vi "Read Encaspulation LEIN Header.vi"(7 "LEIN encapsulated Data and header":u8[](array[numeric]), 11 "error in (no error)":errorcluster) -> (4 "ACK":bool, 6 "SID":u8, 8 "CMD":u8, 10 "LEN":u8, 13 "Data":u8[](array[numeric]), 14 "Data len":i32, 15 "error out":errorcluster)   [LabVIEW 2011]
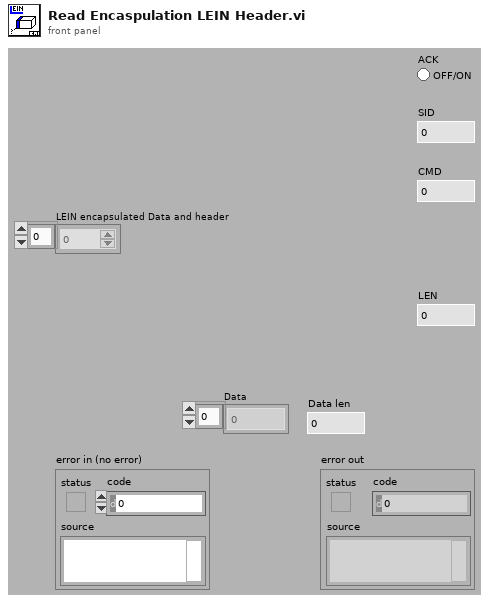
[diagram p1: front panel]
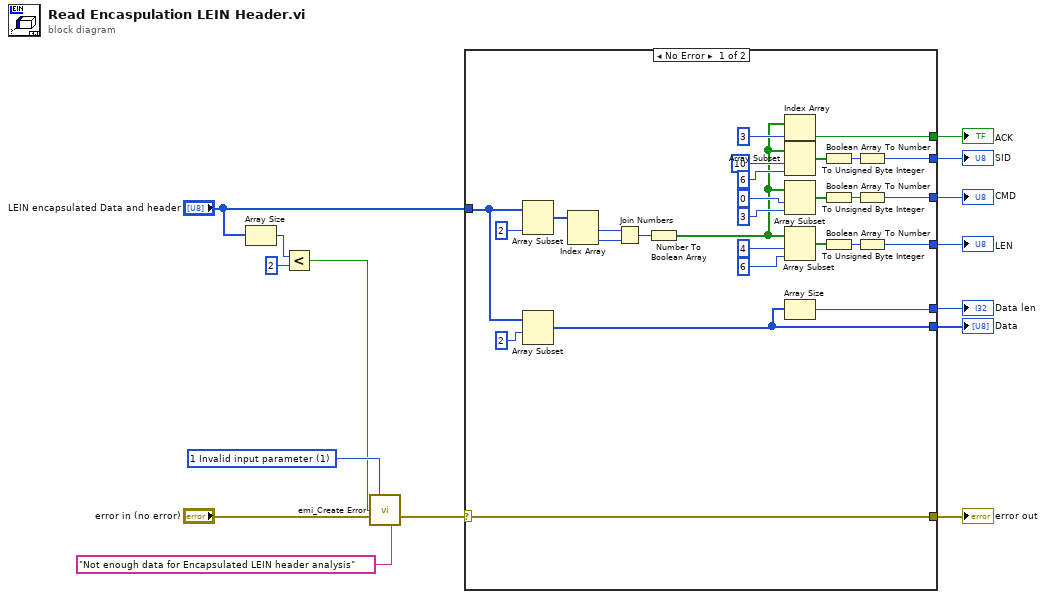
[diagram p0: block diagram]
diagram:
  w5 = 1 items=["0 No Error"=0, "1 Invalid input parameter"=1, "6 Generic file IO "=6, "7 File not Found"=7, "35 Generic Pring Error"=35, "37 Device not Found"=37, "39 Device Unit Error"=39, "40 Could fot Open Device"=40, "42 Generic Error"=42, "52 Unknown Message"=52, "98 Bad File type"=98, "99 Bad File Version"=99, "100 Bad Data in File"=100, "1018 Unspecefied Error"=1018, "1041 Incorrect Password"=1041, "1043 Feature not in this version"=1043, "1109 Unsuported Data type"=1109, "1444 Did not close sucessfully"=1444] ("Error Code")
  n1 = Array Size(array="LEIN encapsulated Data and header") -> (size(s)=w3:i32)
  n2 = Less?(x=w3, y=2) -> (x < y?=w1:bool)
  n3 = call "emi_Create Error.vi"("Error Code"=w5, "Error(T)"=w1, "error in (no error)"="error in (no error)", "Append String(\"\")"="Not enough data for Encapsulated LEIN header analysis" ("Append String(\"\")")) -> ("error out"=w7:errorcluster)  [unwired: 11 in]
  n4 = case shown="No Error" w7 {
    selector: w7 -> [w19 w44]
    tunnel: [w43 _] -> w15
    tunnel: [w42 _] -> w14
    tunnel: [w41 _] -> w13
    tunnel: [w40 _] -> w12
    tunnel: [w39 _] -> w11
    tunnel: "LEIN encapsulated Data and header" -> [w37 _]
    tunnel: [w21 _] -> w10
    tunnel: [w19 w44] -> w6
    frame No Error {
      n5 = Array Subset(array=w37, length=2 ("index")) -> (w36:u8[])  [unwired: 1 in]
      n6 = Array Subset(array=w37, index=2) -> (w21:u8[])  [unwired: 1 in]
      n7 = Index Array(array=w36) -> (element #1=w18:u8, element #2=w17:u8)  [unwired: 2 in]
      n8 = Join Numbers(hi=w18, lo=w17) -> ((hi.lo)=w35:u16)
      n9 = Number To Boolean Array(number=w35) -> (Boolean array=w16:bool[])
      n10 = Index Array(array=w16, index=3) -> (element=w39:bool)
      n11 = Array Subset(array=w16, index=10, length=6) -> (w31:bool[])
      n12 = Array Subset(array=w16, index=0, length=3) -> (w22:bool[])
      n13 = Array Subset(array=w16, index=4, length=6) -> (w32:bool[])
      n14 = Array Size(array=w21) -> (size(s)=w43:i32)
      n15 = Boolean Array To Number(Boolean array=w31) -> (number=w33:u32)
      n16 = Boolean Array To Number(Boolean array=w22) -> (number=w23:u32)
      n17 = Boolean Array To Number(Boolean array=w32) -> (number=w34:u32)
      n18 = To Unsigned Byte Integer(number=w33) -> (unsigned 8bit integer=w40:u8)
      n19 = To Unsigned Byte Integer(number=w23) -> (unsigned 8bit integer=w41:u8)
      n20 = To Unsigned Byte Integer(number=w34) -> (unsigned 8bit integer=w42:u8)
    }
    frame Error {
    }
  }
  "Data len" <- w15
  "LEN" <- w14
  "CMD" <- w13
  "SID" <- w12
  "ACK" <- w11
  "Data" <- w10
  "error out" <- w6
